vi "UserDeletedRow Event Callback.vi"(4 "DataGridView in":refnum<class "DataGridView.lvclass">, 5 "Event Data":cluster{"sender":refnum<k24>, "e":refnum<k24>}, 6 "Control Ref":refnum<k24>, 7 "Event Common Data":T1) -> ()   [LabVIEW 2014, in "DataGrid.lvlib" / "DataGridView.lvclass"]
uses:
  DataGridView/DataGridView.lvclass
  System.Windows.Forms
  Controls/EventsList.ctl
  UserDeletedRow/UserDeletedRow.lvclass
  UserDeletedRow/UserDeletedRow.lvclass/UserDeletedRow.ctl
  UserDeletedRow/Write Row.vi
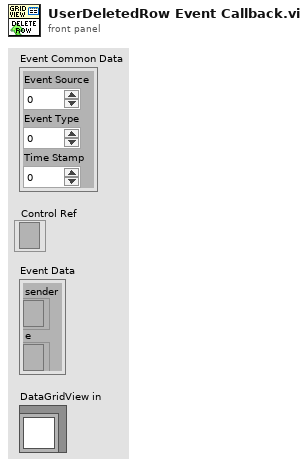
[diagram p1: front panel]
types:
  T1 = cluster{"Event Source":i32, "Event Type":u32, "Time Stamp":u32}
  T2 = typedef "DataGrid.lvlib/DataGridView.lvclass/EventsList.ctl" = enum16{"CellClicked", "CellValueChanged", "KeyDown", "DataError", "UserAddedRow", "UserDeletedRow"}
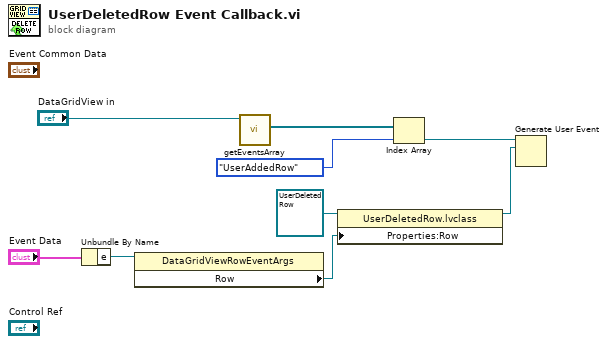
[diagram p0: block diagram]
diagram:
  n1 = Unbundle By Name("Event Data") -> ("e"=w6:refnum<k24>)
  n2 = property class="DataGridViewRowEventArgs"(reference=w6) -> ("Row"=w5:refnum<k24>)  [unwired: 1 in, 2 out]
  n3 = call "getEventsArray.vi"("DataGridView in"="DataGridView in") -> ("userEvents"=w8:refnum<user-event>[])  [unwired: 8 in, 2 out]
  n4 = property class="UserDeletedRow.lvclass"(reference=refnum<class "UserDeletedRow.lvclass"> refnum ("DataGrid.lvlib:UserDeletedRow.lvclass"), "Properties:Row"=w5) -> (reference out=w4:refnum<class "UserDeletedRow.lvclass">)  [unwired: 1 in, 1 out]
  n5 = Index Array(array=w8, index=EventsList."UserAddedRow") -> (element=w7:refnum<user-event>)
  n6 = Generate User Event(user event=w7, event data cluster=w4) -> ()  [unwired: 2 in, 2 out]
